vi "essay_description.vi"(1 "cluster_main_FGV":T1={"Simulation?"=FALSE, "ChanConfigs"=[], "Essay Config"={"HoleDiam"=1.4, "MeanLineDiam"=5.0, "IncF"=0.2, "ElastMod"=207.0, "PoissonMod"=0.3, "RosType"=enum."Tipo A", "Método de análise"=enum."Simplificado 2008", "Pfinal"=0.3, "AStop"=TRUE}, "Directory"=path "", "EssayName"="", "RawFile"=refnum, "InfoFile"=refnum, "DataFile"=refnum, "task"="", "qRecord"=refnum, "qProcess"=refnum} {"ChanConfigs"."GF" min=0.1 max=10.0; "ChanConfigs"."Canal" min=1 max=8}) -> (0 "EssayDescription":string)   [LabVIEW 2016]
uses:
  MainFGV/cluster_main_FGV.ctl
  Config/Channel_config.ctl
  Config/essay_config.ctl
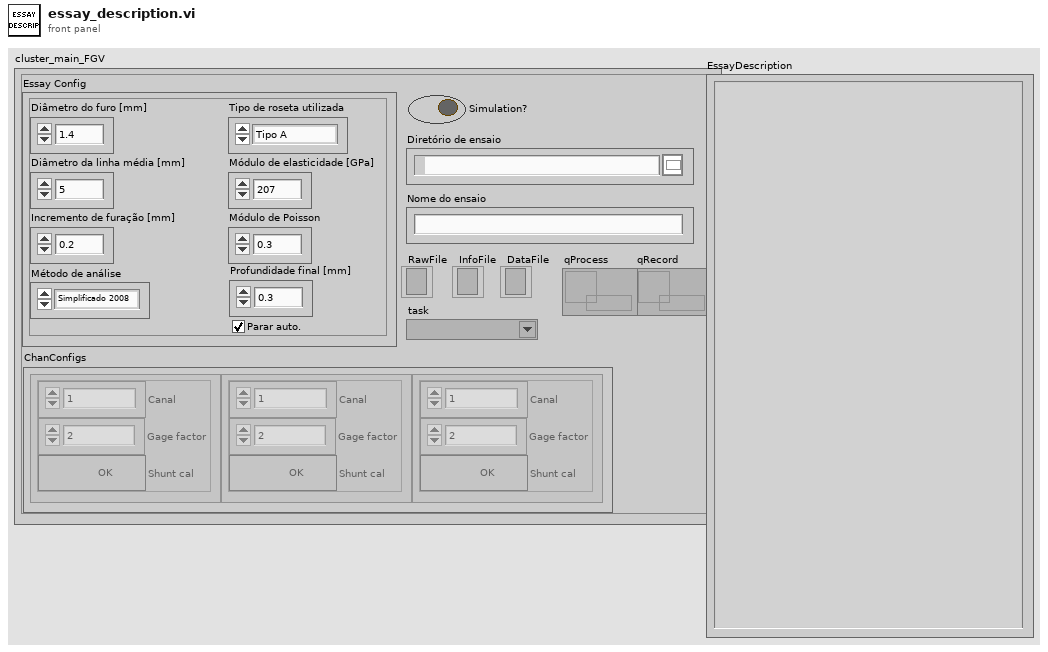
[diagram p1: front panel]
types:
  T1 = typedef "cluster_main_FGV.ctl" = cluster{"Simulation?":bool, "ChanConfigs":T2[], "Essay Config":T3, "Directory":path, "EssayName":string, "RawFile":refnum<file>, "InfoFile":refnum<file>, "DataFile":refnum<file>, "task":refnum<k21>, "qRecord":refnum<queue>, "qProcess":refnum<queue>}
  T2 = typedef "Channel_config.ctl" = cluster{"Canal":i32, "GF":dbl, "SC":bool}
  T3 = typedef "essay_config.ctl" = cluster{"HoleDiam":dbl, "MeanLineDiam":dbl, "IncF":dbl, "ElastMod":dbl, "PoissonMod":dbl, "RosType":enum16{"Tipo A", "Tipo B", "Tipo C"}, "Método de análise":enum16{"Não uniforme 2013", "Simplificado 2013", "Simplificado 2008"}, "Pfinal":dbl, "AStop":bool}
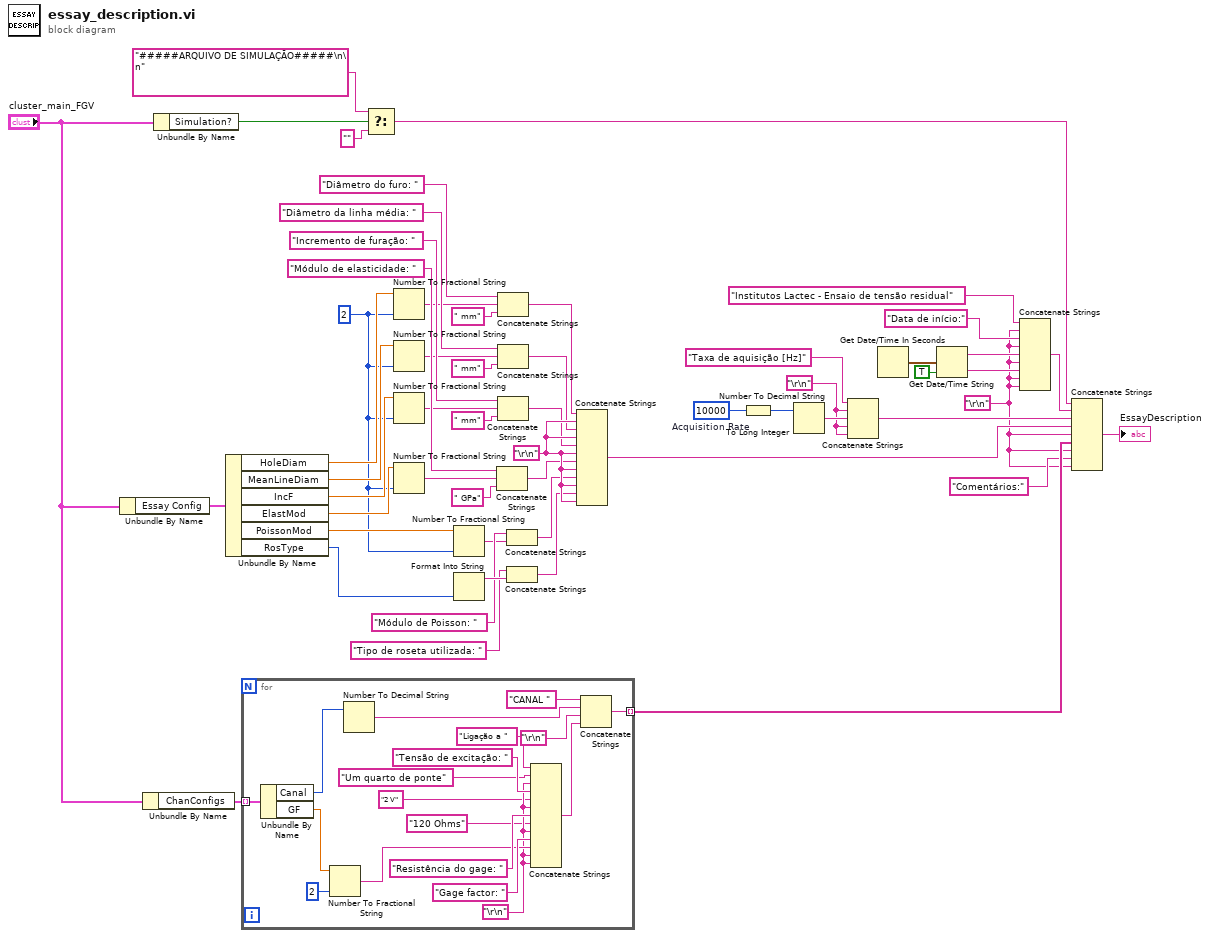
[diagram p0: block diagram]
diagram:
  w7 = i16 2 ("precision (6)")
  w41 = "\r\n"
  w42 = 10000  # Acquisition Rate
  w47 = "\r\n"
  w9 = "\r\n"
  n1 = Unbundle By Name("cluster_main_FGV") -> ("Essay Config"=w12:T3)
  n2 = Unbundle By Name("cluster_main_FGV") -> ("ChanConfigs"=w43:T2[])
  n3 = Unbundle By Name("cluster_main_FGV") -> ("Simulation?"=w4:bool)
  n4 = Unbundle By Name(w12) -> ("HoleDiam"=w14:dbl, "MeanLineDiam"=w19:dbl, "IncF"=w24:dbl, "ElastMod"=w28:dbl, "PoissonMod"=w30:dbl, "RosType"=w32:enum16{"Tipo A", "Tipo B", "Tipo C"})
  n5 = for {
    tunnel: w43 -> [w73] mode=indexing
    tunnel: [w62] -> w44 mode=indexing
    w61 = "\r\n"
    n6 = Unbundle By Name(w73) -> ("Canal"=w60:i32, "GF"=w56:dbl)
    n7 = Number To Fractional String(number=w56, precision (6)=i16 2) -> (F-format string=w67:string)  [unwired: 2 in]
    n8 = Number To Decimal String(number=w60) -> (decimal integer string=w64:string)  [unwired: 1 in]
    n9 = Concatenate Strings("Ligação a " ("string"), "Um quarto de ponte" ("string"), w61, "Tensão de excitação: " ("string"), "2 V" ("string"), w61, "Resistência do gage: " ("string"), "120 Ohms" ("string"), w61, "Gage factor: " ("string"), w67, w61, w61) -> (w65:string)
    n10 = Concatenate Strings("CANAL " ("string"), w64, "\r\n", w65) -> (w62:string)
  }
  n11 = Select(t="#####ARQUIVO DE SIMULAÇÃO#####\n\n" ("string"), s=w4, f="") -> (s? t:f=w1:string)
  n12 = Number To Fractional String(number=w14, precision (6)=w7) -> (F-format string=w15:string)  [unwired: 2 in]
  n13 = Number To Fractional String(number=w19, precision (6)=w7) -> (F-format string=w18:string)  [unwired: 2 in]
  n14 = Number To Fractional String(number=w24, precision (6)=w7) -> (F-format string=w22:string)  [unwired: 2 in]
  n15 = Number To Fractional String(number=w28, precision (6)=w7) -> (F-format string=w26:string)  [unwired: 2 in]
  n16 = Number To Fractional String(number=w30, precision (6)=w7) -> (F-format string=w29:string)  [unwired: 2 in]
  n17 = Format Into String(w32) -> (resulting string=w34:string)  [unwired: 3 in, 1 out]
  n18 = Concatenate Strings("Módulo de elasticidade: " ("string"), w26, " GPa" ("string")) -> (w38:string)
  n19 = Concatenate Strings("Diâmetro do furo: " ("string"), w15, " mm" ("string")) -> (w35:string)
  n20 = Concatenate Strings("Diâmetro da linha média: " ("string"), w18, " mm" ("string")) -> (w36:string)
  n21 = Concatenate Strings("Incremento de furação: " ("string"), w22, " mm" ("string")) -> (w37:string)
  n22 = Concatenate Strings("Módulo de Poisson: " ("string"), w29) -> (w39:string)
  n23 = Concatenate Strings("Tipo de roseta utilizada: " ("string"), w34) -> (w40:string)
  n24 = Concatenate Strings(w35, w41, w36, w41, w37, w41, w38, w41, w39, w41, w40, w41) -> (w11:string)
  n25 = To Long Integer(number=w42) -> (32bit integer=w50:i32)
  n26 = Number To Decimal String(number=w50) -> (decimal integer string=w49:string)  [unwired: 1 in]
  n27 = Concatenate Strings("Taxa de aquisição [Hz]" ("string"), w47, w49, w47, w47) -> (w46:string)
  n28 = Get Date/Time In Seconds() -> (seconds since 1Jan1904=w55:timestamp)
  n29 = Get Date/Time String(seconds (now)=w55, want seconds? (F)=TRUE) -> (date string=w54:string, time string=w53:string)  [unwired: 1 in]
  n30 = Concatenate Strings("Institutos Lactec - Ensaio de tensão residual" ("string"), w9, "Data de início:" ("string"), w9, w54, w9, w53, w9, w9) -> (w51:string)
  n31 = Concatenate Strings(w1, w51, w46, w11, w9, w44, w9, "Comentários:" ("string"), w9) -> (→"EssayDescription":string)
